vi "Byte_buffer.vi"(9 "byte queue":refnum<queue>, 11 "reference":refnum<visa-resource-name>) -> (1 "Bytes at Port":u32, 3 "byte queue out":refnum<queue>)   [LabVIEW 2017]
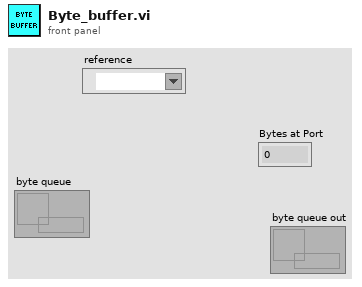
[diagram p1: front panel]
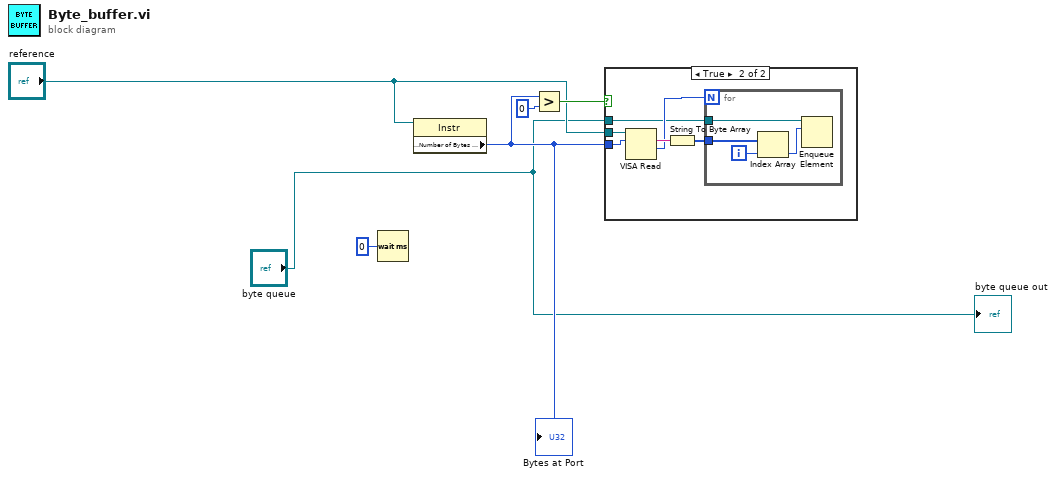
[diagram p0: block diagram]
diagram:
  n1 = Wait (ms)(milliseconds to wait=u32 0) -> ()  [unwired: 1 out]
  n2 = property class="Instr"(reference="reference") -> ("Serial Settings:Number of Bytes at Serial Port"=w4:u32)  [unwired: 1 in, 2 out]
  "Bytes at Port" <- w4
  n3 = Greater?(x=w4, y=u32 0) -> (0:w5:bool)
  n4 = case shown="True" w5 {
    tunnel: w4 -> [_ w12]
    tunnel: "byte queue" -> [_ w9]
    tunnel: "reference" -> [_ w7]
    frame False {
    }
    frame True {
      n5 = VISA Read(VISA resource name=w7, byte count=w12) -> (read buffer=w11:string, return count=w10:u32)  [unwired: 1 in, 2 out]
      n6 = String To Byte Array(string=w11) -> (unsigned byte array=w8:u8[])
      n7 = for {
        N: w10 -> [_]
        tunnel: w9 -> [w16]
        tunnel: w8 -> [w15]
        i -> [w14]
        n8 = Index Array(array=w15, index=w14) -> (element=w13:u8)
        n9 = Enqueue Element(queue=w16, element=w13) -> ()  [unwired: 2 in, 3 out]
      }
    }
  }
  "byte queue out" <- "byte queue"
